vi "Send Message.vi"   [LabVIEW 2015, in "Execution.lvclass"]
uses:
  Execution.lvclass
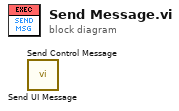
[diagram p0: block diagram]
diagram:
  n1 = call "Send UI Message.vi"() -> ()  [unwired: 11 in, 1 out]
  n2 = call "Send Control Message.vi"() -> ()  [unwired: 11 in, 1 out]
